vi "Actor Core.vi"(8 "error in":errorcluster, 11 "Watchdog in":refnum<class "Watchdog.lvclass">) -> (0 "error out":errorcluster, 3 "Actor out":refnum<class "Actor.lvclass">)   [LabVIEW 2015, in "Watchdog Actor.lvlib" / "Watchdog.lvclass"]
doc: "(<B>Filename</B>: Actor Framework.lvlib:Actor.lvclass:Actor Core.vi)\n\nReceives messages to the actor, reacts to them, and initiates any error handling that may shut the actor down.\n\nDescendant classes may override this VI to append parallel tasks for the actor to complete while it handles messages. Overrides use the Call Parent Method node."
uses:
  Watchdog.lvclass
  <vilib>/ActorFramework/Actor/Actor.lvclass
  Watchdog.lvclass/Watchdog.ctl
  <vilib>/Modbus/master/Modbus Master.lvclass
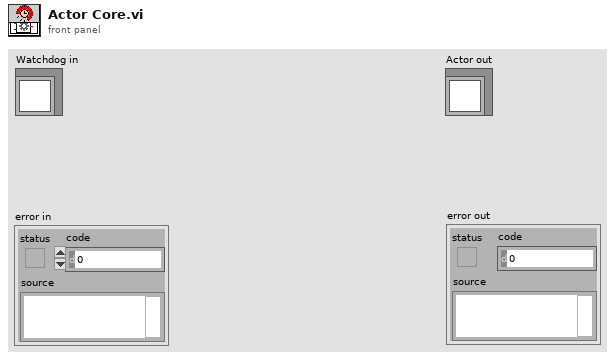
[diagram p1: front panel]
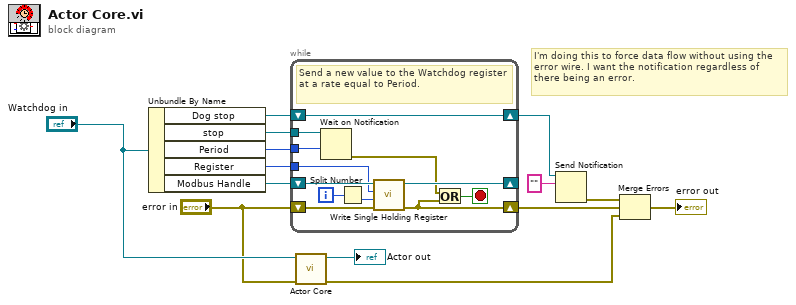
[diagram p0: block diagram]
diagram:
  # "I'm doing this to force data flow without using the error wire. I want the notification regardless of there being an error."
  n1 = Unbundle By Name("Watchdog in") -> ("Dog stop"=w2:refnum<notifier>, "stop"=w12:refnum<notifier>, "Period"=w8:i32, "Register"=w9:u16, "Modbus Handle"=w5:refnum<class "Modbus Master.lvclass">)
  n2 = while {
    tunnel: w12 -> [w21]
    tunnel: w8 -> [w20]
    tunnel: w9 -> [w19]
    shift-right: [w23] -> w7
    shift-left: "error in" -> [w26]
    shift-right: [w24] -> _
    shift-left: w5 -> [w25]
    shift-right: [w16] -> w1
    shift-left: w2 -> [w16]
    i -> [w17]
    stop <- w18 stop-if-true
    # "Send a new value to the Watchdog register at a rate equal to Period."
    n3 = Wait on Notification(notifier=w21, timeout in ms (-1)=w20) -> (error out=w15:errorcluster)  [unwired: 2 in, 3 out]
    n4 = Split Number(x=w17) -> (lo(x)=w22:u16)  [unwired: 1 out]
    n5 = call-dynamic "Write Single Holding Register.vi"("error in (no error)"=w26, "holding register value"=w22, "address"=w19, "Modbus master in"=w25) -> ("error out"=w23:errorcluster, "Modbus master out"=w24:refnum<class "Modbus Master.lvclass">)  [unwired: 6 in]
    n6 = Or(x=w15, y=w23) -> (x .or. y?=w18:bool)
  }
  n7 = call-parent "Actor Core.vi"("error in"="error in", "Actor in"="Watchdog in") -> ("error out"=w14:errorcluster, "Actor out"=→"Actor out":refnum<class "Actor.lvclass">)  [unwired: 8 in]
  n8 = Send Notification(notification="", notifier=w1) -> (error out=w4:errorcluster)  [unwired: 1 in, 1 out]
  n9 = Merge Errors(w4, w7, w14) -> (→"error out":errorcluster)
